vi "ReadScriptFile.vi"(8 "error in (no error)":errorcluster, 11 "File":path) -> (0 "error out":errorcluster, 3 "Script":string[][](array[string]), 5 "#Rows":i32)   [LabVIEW 2011]
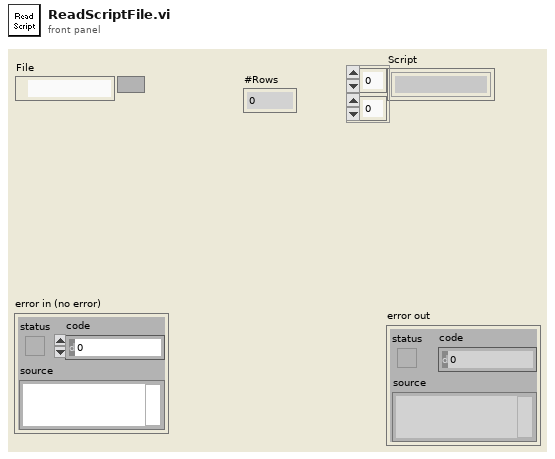
[diagram p1: front panel]
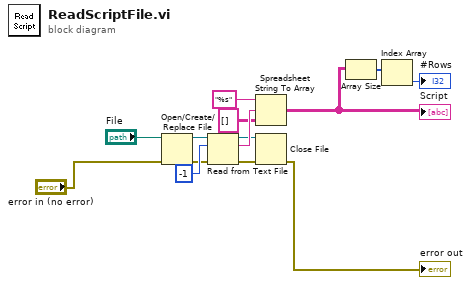
[diagram p0: block diagram]
diagram:
  n1 = Open/Create/Replace File(file path (use dialog)="File", error in="error in (no error)") -> (refnum out=w6:refnum<file>, error out=w7:errorcluster)  [unwired: 5 out]
  n2 = Read from Text File(file (use dialog)=w6, count=-1, error in=w7) -> (refnum out=w5:refnum<file>, text=w11:string, error out=w8:errorcluster)  [unwired: 2 out]
  n3 = Spreadsheet String To Array(format string="%s" ("spreadsheet string"), spreadsheet string=w11, array type (2D Dbl)=string[][] [] ("Item Names")) -> (array=w1:string[][])  [unwired: 1 out]
  "Script" <- w1
  n4 = Close File(refnum=w5, error in=w8) -> (error out=→"error out":errorcluster)  [unwired: 1 out]
  n5 = Array Size(array=w1) -> (size(s)=w13:i32[])
  n6 = Index Array(array=w13) -> (element=→"#Rows":i32)  [unwired: 1 in]
